vi "lvgitSave Configuration Settings to XML.vi"(8 "error in (no error)":errorcluster, 11 "User Configuration":T1={"Hardware Configuration"={"HW Refnum <Replace Me>"="", "Signal Type <Replace Me>"=enum."Sine Wave"}, "Analysis Configuration"={"Statistics"=TRUE}, "New Data Behavior"=enum."Replace"}) -> (0 "error out":errorcluster)   [LabVIEW 2012]
doc: "Saves the user-specified configuration data to an XML file. This is used to remember settings between executions."
uses:
  controls/lvgitUser Specified Data.ctl
  controls/lvgitHW Configuration.ctl
  controls/lvgitSimulated Signal Type.ctl
  controls/lvgitAnalysis Configuration.ctl
  controls/lvgitNew Data Behavior.ctl
  <vilib>/Utility/xml.llb/Write to XML File(string).vi
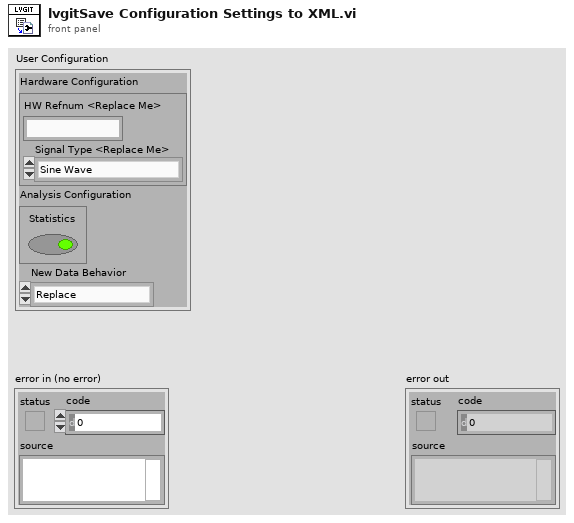
[diagram p1: front panel]
types:
  T1 = typedef "lvgitUser Specified Data.ctl" = cluster{"Hardware Configuration":T2, "Analysis Configuration":T4, "New Data Behavior":T5}
  T2 = typedef "lvgitHW Configuration.ctl" = cluster{"HW Refnum <Replace Me>":string, "Signal Type <Replace Me>":T3}
  T3 = typedef "lvgitSimulated Signal Type.ctl" = enum16{"Sine Wave", "Square Wave"}
  T4 = typedef "lvgitAnalysis Configuration.ctl" = cluster{"Statistics":bool}
  T5 = typedef "lvgitNew Data Behavior.ctl" = enum16{"Replace", "Overlay", "Append"}
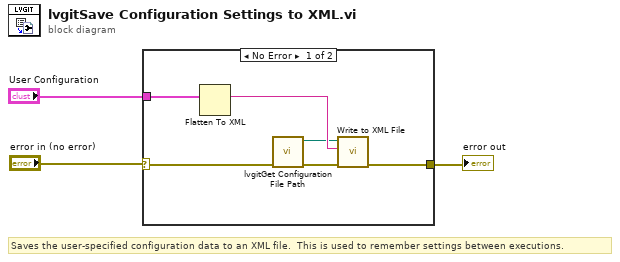
[diagram p0: block diagram]
diagram:
  # "Saves the user-specified configuration data to an XML file.  This is used to remember settings between executions."
  n1 = case shown="No Error" "error in (no error)" {
    selector: "error in (no error)" -> [w5 w10]
    tunnel: [w7 w10] -> w2
    tunnel: "User Configuration" -> [w9 _]
    frame No Error {
      n2 = Flatten To XML(anything=w9) -> (xml string=w8:string)
      n3 = call "lvgitGet Configuration File Path.vi"("error in (no error)"=w5) -> ("error out"=w4:errorcluster, "XML File Path"=w6:path)  [unwired: 9 in]
      n4 = call-poly <vilib>:"Write to XML File.vi"("error in (no error)"=w4, "XML Input"=w8, "XML File Path"=w6) -> ("error out"=w7:errorcluster)  [unwired: 6 in, 2 out]
    }
    frame Error {
    }
  }
  "error out" <- w2
